vi "Configuration File Get VeriStand Application Path.vi"(8 "error in (no error)":errorcluster) -> (0 "error out":errorcluster, 2 "Found?":bool, 3 "VeriStand Application Path":path)   [LabVIEW 2020, in "ni-veristand-steps-runtime-lib.lvlib"]
uses:
  ni-veristand-steps-runtime-lib.lvlib
  <vilib>/Utility/config.llb/Read Key (String).vi
  <vilib>/Utility/config.llb/NI_LVConfig.lvlib
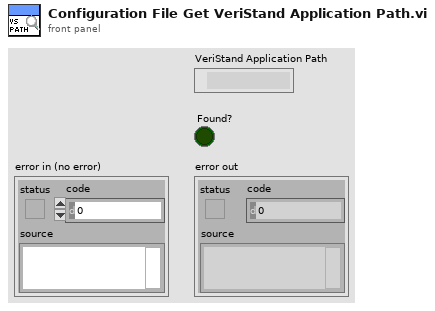
[diagram p1: front panel]
types:
  T1 = typedef "NI_LVConfig.lvlib/Config Data RefNum.ctl" = refnum<k1>
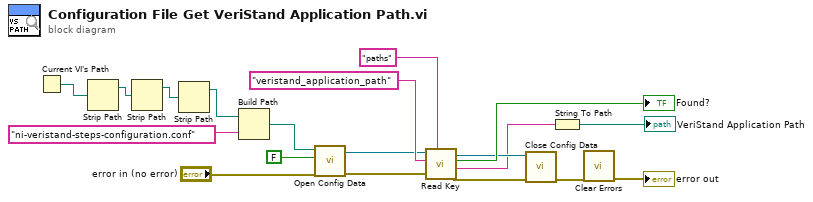
[diagram p0: block diagram]
diagram:
  n1 = Current VI's Path() -> (path=w18:path)
  n2 = Strip Path(path=w18) -> (stripped path=w4:path)  [unwired: 1 out]
  n3 = Strip Path(path=w4) -> (stripped path=w3:path)  [unwired: 1 out]
  n4 = Strip Path(path=w3) -> (stripped path=w2:path)  [unwired: 1 out]
  n5 = Build Path(base path=w2, name or relative path="ni-veristand-steps-configuration.conf") -> (appended path=w1:path)
  n6 = call <vilib>:"Open Config Data.vi"("error in (no error)"="error in (no error)", "create file if necessary (T)"=FALSE, "configuration file path"=w1) -> ("error out"=w13:errorcluster, "refnum"=w12:T1)  [unwired: 6 in, 1 out]
  n7 = call-poly <vilib>:"Read Key.vi"("section"="paths", "error in (no error)"=w13, "key"="veristand_application_path", "refnum"=w12) -> ("error out"=w17:errorcluster, "value"=w6:string, "found?"=→"Found?":bool, "refnum out"=w16:T1)  [unwired: 4 in]
  n8 = call <vilib>:"Close Config Data.vi"("error in (no error)"=w17, "refnum"=w16) -> ("error out"=w8:errorcluster)  [unwired: 8 in, 1 out]
  n9 = String To Path(string=w6) -> (path=→"VeriStand Application Path":path)
  n10 = call <vilib>:"Clear Errors.vi"("error in (no error)"=w8) -> ("error out"=→"error out":errorcluster)  [unwired: 5 in, 1 out]
